vi "Invert Joystick Y Axes.vi"(1 "Axes in":T1) -> (0 "Axes out":T1)   [LabVIEW 2013]
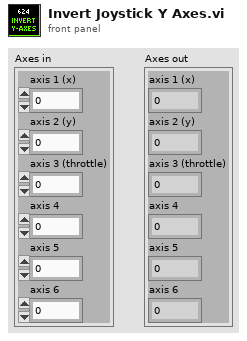
[diagram p1: front panel]
types:
  T1 = cluster{"axis 1 (x)":dbl, "axis 2 (y)":dbl, "axis 3 (throttle)":dbl, "axis 4":dbl, "axis 5":dbl, "axis 6":dbl}
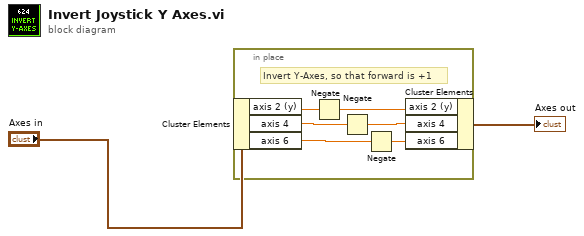
[diagram p0: block diagram]
diagram:
  n1 = in-place {
    # "Invert Y-Axes, so that forward is +1"
    n2 = in-place-cluster #1("Axes in") -> ("axis 2 (y)"=w8:dbl, "axis 4"=w6:dbl, "axis 6"=w4:dbl)
    n3 = Negate(x=w8) -> (-x=w7:dbl)
    n4 = Negate(x=w6) -> (-x=w5:dbl)
    n5 = Negate(x=w4) -> (-x=w3:dbl)
    n6 = in-place-cluster #1("axis 2 (y)"=w7, "axis 4"=w5, "axis 6"=w3) -> (→"Axes out":T1)
  }
